vi "5p1_HW_Task1_fishele.vi"() -> ()   [LabVIEW 2021]
uses:
  <vilib>/express/express arith-compare/Formula/XNode/ExpressFormulaBlockNode.xnode
panel:
  out "ERROR LOG":string="All inputs look good"
  out "Attraction":string="One negative"
  out "Force (Newtons)":dbl format="%#_30f"
  in  "D (meters)":dbl
  in  "Q2 (Coulombs)":dbl
  in  "Q1 (Coulombs)":dbl
  # "Using Coulomb's Law to Determine Attraction and Force"
  # "Input"
  # "Output"
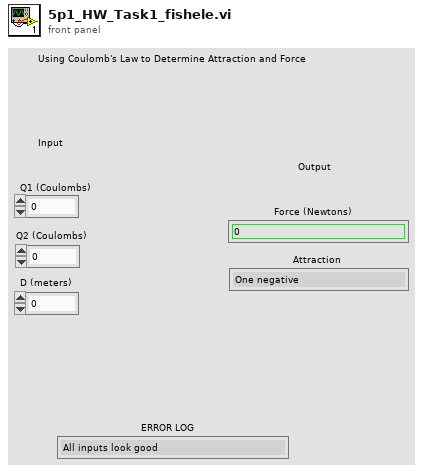
[diagram p1: front panel]
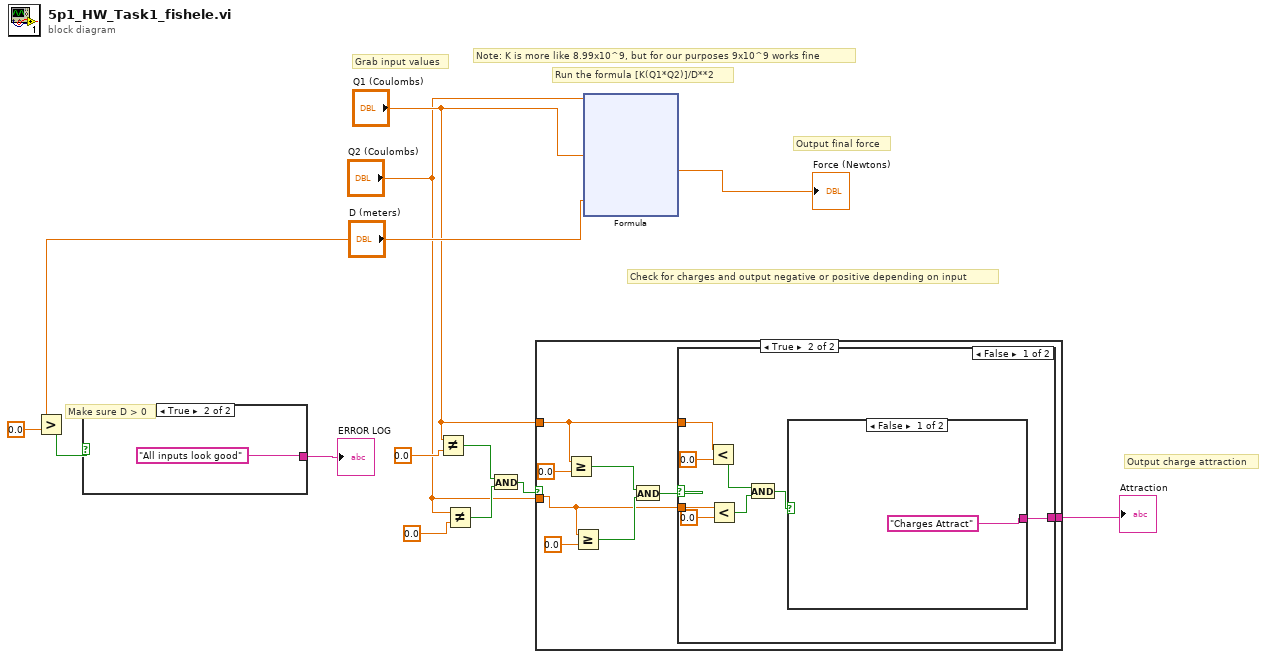
[diagram p0: block diagram]
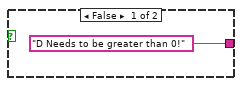
[diagram p2: hidden frame]
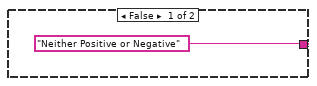
[diagram p3: hidden frame]
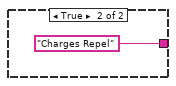
[diagram p4: hidden frame]
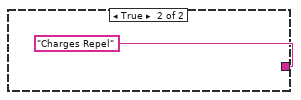
[diagram p5: hidden frame]
diagram:
  # "Make sure D > 0"
  # "Output charge attraction"
  # "Note: K is more like 8.99x10^9, but for our purposes 9x10^9 works fine"
  # "Output final force"
  # "Grab input values"
  # "Run the formula [K(Q1*Q2)]/D**2"
  # "Check for charges and output negative or positive depending on input"
  n1 = Greater?(x="D (meters)", y=0.0) -> (0:w4:bool)
  n2 = case shown="True" w4 {
    tunnel: ["D Needs to be greater than 0!" "All inputs look good"] -> w3
    frame False {
    }
    frame True {
    }
  }
  "ERROR LOG" <- w3
  n3 = Not Equal?(x="Q1 (Coulombs)", y=0.0) -> (x != y?=w9:bool)
  n4 = Not Equal?(x="Q2 (Coulombs)", y=0.0) -> (x != y?=w8:bool)
  n5 = And(x=w9, y=w8) -> (x .and. y?=w7:bool)
  n6 = case shown="True" w7 {
    tunnel: ["Neither Positive or Negative" w19] -> w12
    tunnel: "Q1 (Coulombs)" -> [_ w18]
    tunnel: "Q2 (Coulombs)" -> [_ w17]
    frame False {
    }
    frame True {
      n7 = Greater Or Equal?(x=w18, y=0.0) -> (x >= y?=w22:bool)
      n8 = Greater Or Equal?(x=w17, y=0.0) -> (x >= y?=w21:bool)
      n9 = And(x=w22, y=w21) -> (x .and. y?=w20:bool)
      n10 = case shown="False" w20 {
        tunnel: [w28 "Charges Repel"] -> w19
        tunnel: w18 -> [w26 _]
        tunnel: w17 -> [w25 _]
        frame False {
          n11 = Less?(x=w26, y=0.0) -> (x < y?=w30:bool)
          n12 = Less?(x=w25, y=0.0) -> (x < y?=w29:bool)
          n13 = And(x=w30, y=w29) -> (x .and. y?=w27:bool)
          n14 = case shown="False" w27 {
            tunnel: ["Charges Attract" "Charges Repel"] -> w28
            frame False {
            }
            frame True {
            }
          }
        }
        frame True {
        }
      }
    }
  }
  "Attraction" <- w12
  n15 = xnode "Formula"("Q1"="Q1 (Coulombs)", "Q2"="Q2 (Coulombs)", "D"="D (meters)") -> ("Result"=→"Force (Newtons)":dbl)  [unwired: 1 in, 1 out]
